vi "grain_coords_to_a_b.vi"(8 "Error In":errorcluster, 9 "Parameters":T1, 10 "y":dbl, 11 "x":dbl) -> (0 "Error Out":errorcluster, 2 "b":dbl, 3 "a":dbl)   [LabVIEW 2019]
doc: "Takes grain pixel coordinates and the center of rotation to turn the grain coordinates into a and b for further calculations."
uses:
  parameters_cluster_typedef.ctl
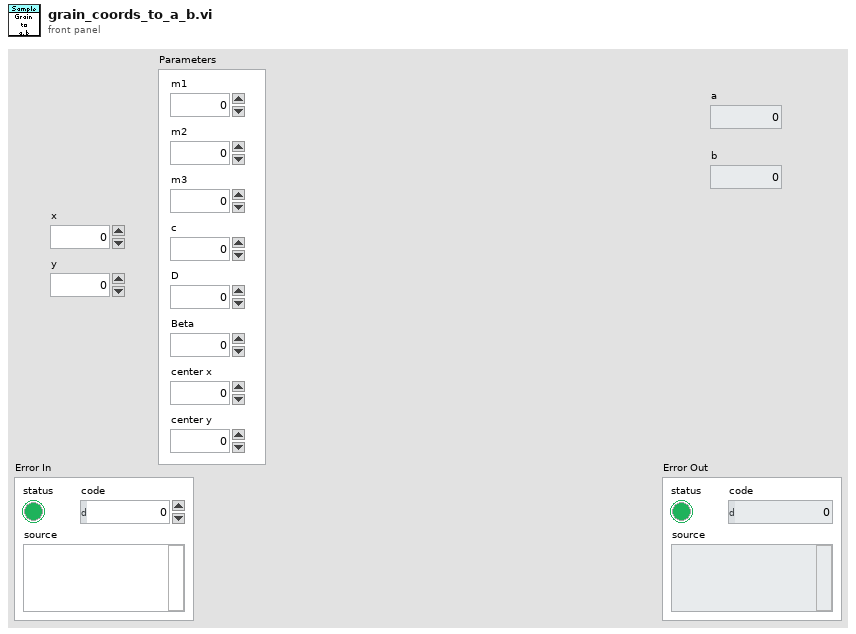
[diagram p1: front panel]
types:
  T1 = typedef "parameters_cluster_typedef.ctl" = cluster{"m1":dbl, "m2":dbl, "m3":dbl, "c":dbl, "D":dbl, "Beta":dbl, "center x":dbl, "center y":dbl}
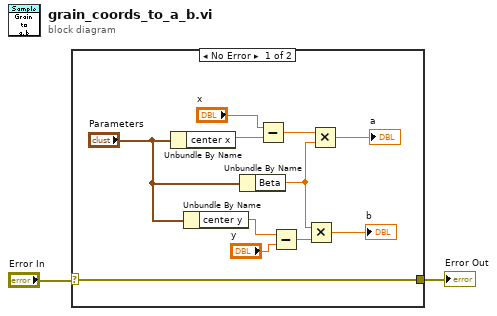
[diagram p0: block diagram]
diagram:
  n1 = case shown="No Error" "Error In" {
    selector: "Error In" -> [w13 w14]
    tunnel: [w13 w14] -> w1
    frame No Error {
      n2 = Unbundle By Name("Parameters") -> ("center x"=w12:dbl)
      n3 = Unbundle By Name("Parameters") -> ("center y"=w9:dbl)
      n4 = Unbundle By Name("Parameters") -> ("Beta"=w5:dbl)
      n5 = Subtract(x="x", y=w12) -> (x-y=w7:dbl)
      n6 = Subtract(x=w9, y="y") -> (x-y=w6:dbl)
      n7 = Multiply(x=w5, y=w6) -> (x*y=→"b":dbl)
      n8 = Multiply(x=w7, y=w5) -> (x*y=→"a":dbl)
    }
    frame Error {
    }
  }
  "Error Out" <- w1
